vi "Convert Device Units to Position Units (FW7).vi"(9 "Microstep Size (0)":dbl, 10 "Units (0: microsteps)":u16(ring) items=["microsteps", "microns", "millimeters", "inches", "degrees"], 11 "Device Position (0)":i64) -> (3 "Position":dbl)   [LabVIEW 2021, in "Zaber A Series.lvlib"]
doc: "Helper to convert device-specific position units to standard units of measure.\n\nPass in a position measurement from a device and a unit to convert to. The output will be the measurement converted to the selected units.\n\nIf you select a unit other than microsteps, you must also provide the Microstep Size conversion factor from microsteps to micrometers (for linear devices) or degrees (for rotary devices), which can be found in your device manual."
uses:
  Zaber A Series.lvlib
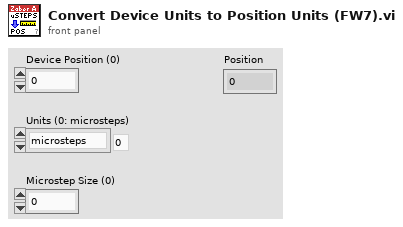
[diagram p1: front panel]
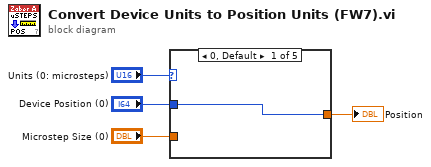
[diagram p0: block diagram]
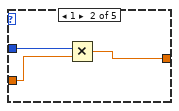
[diagram p2: hidden frame]
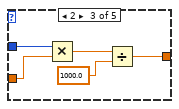
[diagram p3: hidden frame]
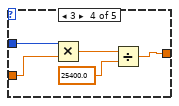
[diagram p4: hidden frame]
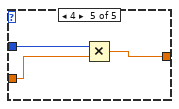
[diagram p5: hidden frame]
diagram:
  n1 = case shown="0, Default" "Units (0: microsteps)" {
    tunnel: "Microstep Size (0)" -> [_ w7 w12 w15 w20]
    tunnel: "Device Position (0)" -> [w5 w8 w13 w16 w21]
    tunnel: [w5 w6 w9 w14 w19] -> w1
    frame 0, Default {
    }
    frame 1 {
      n2 = Multiply(x=w8, y=w7) -> (x*y=w6:dbl)
    }
    frame 2 {
      n3 = Multiply(x=w13, y=w12) -> (x*y=w11:dbl)
      n4 = Divide(x=w11, y=1000.0) -> (x/y=w9:dbl)
    }
    frame 3 {
      n5 = Multiply(x=w16, y=w15) -> (x*y=w17:dbl)
      n6 = Divide(x=w17, y=25400.0) -> (x/y=w14:dbl)
    }
    frame 4 {
      n7 = Multiply(x=w21, y=w20) -> (x*y=w19:dbl)
    }
  }
  "Position" <- w1
